vi "Do.vi"(8 "error in (no error)":errorcluster, 10 "Actor in":refnum<class "Actor.lvclass">, 11 "Update-PV Msg":refnum<class "Update-PV Msg.lvclass">) -> (0 "error out":errorcluster, 2 "Actor out":refnum<class "Actor.lvclass">)   [LabVIEW 2016, in "CS++OPCUAInterface.lvlib" / "Update-PV Msg.lvclass"]
doc: "(<B>Filename</B>: Actor Framework.lvlib:Message.lvclass:Do.vi)\n\nDefines what a message does when it is received by an actor. Generally, a message instructs an actor to invoke one of its methods.\n\nBy default, this method does nothing. A child class must override it to define behavior. Create a child class by using the Actor Framework Message Maker dialog box."
uses:
  Update-PV Msg.lvclass
  C:/User/Brand/LVP/CSPP-Dev/Packages/CSPP_Core/Actors/CS++PVMonitor Messages/CS++PVUpdate Msg/CS++PVUpdate Msg.lvclass
  <vilib>/ActorFramework/Actor/Actor.lvclass
  CS++OPCUAInterface/CS++OPCUAInterface.lvclass
  C:/Program Files (x86)/National Instruments/LabVIEW 2016/vi.lib/ActorFramework/Actor/Actor.lvclass
  CSPP_Core/Actors/CS++PVMonitor Messages/CS++PVUpdate Msg/CS++PVUpdate Msg.lvclass/CS++PVUpdate Msg.ctl
  CSPP_Core/Classes/CS++ProcessVariables/ProcessVariable/PV.lvclass
  CSPP_Core/Actors/CS++PVMonitor Messages/CS++PVUpdate Msg/CS++PVUpdate Msg.lvclass
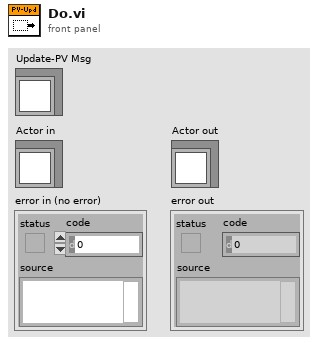
[diagram p1: front panel]
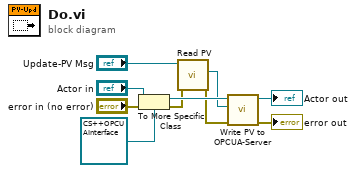
[diagram p0: block diagram]
diagram:
  n1 = To More Specific Class(target class=refnum<class "CS++OPCUAInterface.lvclass"> refnum ("CS++OPCUAInterface.lvlib:CS++OPCUAInterface.lvclass"), reference="Actor in", error in="error in (no error)") -> (specific class reference=w7:refnum<class "CS++OPCUAInterface.lvclass">, error out=w5:errorcluster)
  n2 = call "Read PV.vi"("error in (no error)"=w5, "CS++PVUpdate Msg in"="Update-PV Msg") -> ("error out"=w3:errorcluster, "PV"=w4:refnum<class "PV.lvclass">)  [unwired: 7 in, 1 out]
  n3 = call "Write PV to OPCUA-Server.vi"("Error In"=w3, "PV"=w4, "CS++OPCUAInterface in"=w7) -> ("Error Out"=→"error out":errorcluster, "CS++OPCUAInterface out"=→"Actor out":refnum<class "CS++OPCUAInterface.lvclass">)  [unwired: 7 in]
